vi "Save Message Folder.vi"(8 "error in (no error)":errorcluster, 9 ".proto Path":path, 10 "Output Folder":path) -> (0 "error out":errorcluster)   [LabVIEW 2020, in "LV-Protoc.lvlib" / "LV-Protoc.lvclass"]
uses:
  LV-Protoc.lvclass
  lv-cdm/CDM-Config/Config-JSON/Config-JSON.lvclass
  C:/dev/lv20CE/relink/lv-cdm/CDM-Config/Config Storage/Config Storage.lvclass
  lv-cdm/CDM-Config/Config Element/Write Variant Value.vi
  lv-cdm/CDM-Config/Config Manager/Config Manager.lvclass
  lv-cdm/CDM-Config/Config Element/Config Element.lvclass
  LV-Protoc.lvclass/LV-Protoc.ctl
  lv-cdm/CDM-Config/Config Storage/Config Storage.lvclass
  lv-cdm/CDM-Config/CDM-Config.lvlib
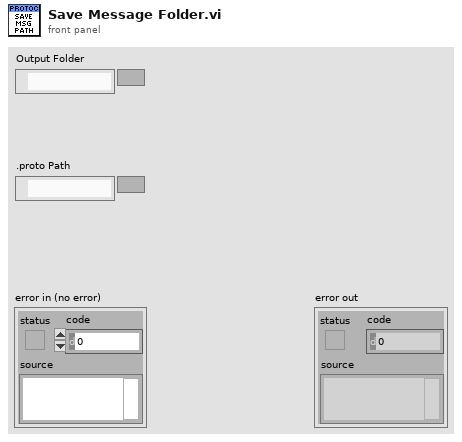
[diagram p1: front panel]
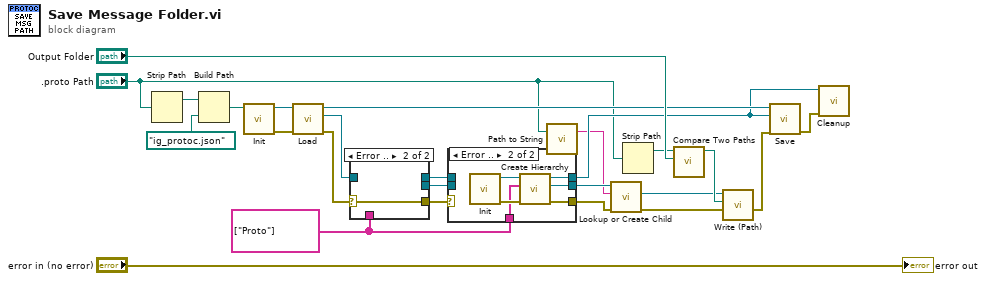
[diagram p0: block diagram]
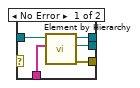
[diagram p2: hidden frame]
diagram:
  w11 = string[] ["Proto"] ("Hierarchy")
  n1 = Strip Path(path=".proto Path") -> (stripped path=w19:path)  [unwired: 1 out]
  n2 = Build Path(base path=w19, name or relative path=path "ig_protoc.json") -> (appended path=w23:path)
  n3 = call "Init.vi"("Path"=w23) -> ("error out"=w22:errorcluster, "Config-JSON out"=w21:refnum<class "Config-JSON.lvclass">)  [unwired: 9 in]
  n4 = call "Load.vi"("error in (no error)"=w22, "Config Storage in"=w21) -> ("error out"=w20:errorcluster, "Config"=w14:refnum<class "Config Manager.lvclass">, "Config Storage out"=w16:refnum<class "Config-JSON.lvclass">)  [unwired: 7 in]
  n5 = case shown="Error .." w20 {
    selector: w20 -> [_ w31]
    tunnel: w14 -> [w30 _]
    tunnel: w11 -> [w29 _]
    tunnel: [w28 _] -> w9
    tunnel: [w27 w31] -> w10
    tunnel: [w26 _] -> w6
    frame No Error {
      n6 = call "Element by Hierarchy.vi"("Hierarchy"=w29, "Config Manager in"=w30) -> ("error out"=w27:errorcluster, "Config Element"=w28:refnum<class "Config Element.lvclass">, "Config Manager out"=w26:refnum<class "Config Manager.lvclass">)  [unwired: 7 in]
    }
    frame Error {
    }
  }
  n7 = case shown="Error .." w10 {
    selector: w10 -> [w33 _]
    tunnel: [w34 w40] -> w13
    tunnel: [w33 w39] -> w12
    tunnel: w11 -> [_ w36]
    tunnel: w9 -> [w34 _]
    tunnel: w6 -> [w32 _]
    tunnel: [w32 w35] -> w5
    frame No Error {
    }
    frame Error {
      n8 = call "Init.vi"() -> ("error out"=w37:errorcluster, "Config Manager out"=w38:refnum<class "Config Manager.lvclass">)  [unwired: 10 in]
      n9 = call "Create Hierarchy.vi"("error in (no error)"=w37, "Hierarchy"=w36, "Config Manager in"=w38) -> ("error out"=w39:errorcluster, "Leaf Element"=w40:refnum<class "Config Element.lvclass">, "Config Manager out"=w35:refnum<class "Config Manager.lvclass">)  [unwired: 6 in]
    }
  }
  n10 = call "Path to String.vi"("Path"=".proto Path") -> ("Path String"=w3:string)  [unwired: 2 in]
  n11 = call "Lookup or Create Child.vi"("error in (no error)"=w12, "Name"=w3, "Config Element in"=w13) -> ("error out"=w7:errorcluster, "Child"=w8:refnum<class "Config Element.lvclass">)  [unwired: 5 in, 2 out]
  n12 = Strip Path(path=".proto Path") -> (stripped path=w4:path)  [unwired: 1 out]
  n13 = call <vilib>:"Compare Two Paths.vi"("Path 2"="Output Folder", "Path 1"=w4) -> ("Relative Path from 1 to 2"=w17:path)  [unwired: 6 in, 3 out]
  n14 = call "Write (Path).vi"("error in (no error)"=w7, "Path Value"=w17, "Config Element in"=w8) -> ("error out"=w15:errorcluster)  [unwired: 7 in, 1 out]
  n15 = call "Save.vi"("error in (no error)"=w15, "Config"=w5, "Config Storage in"=w16) -> ("error out"=w1:errorcluster)  [unwired: 7 in, 1 out]
  n16 = call "Cleanup.vi"("error in (no error)"=w1, "Config Manager in"=w5) -> ()  [unwired: 9 in, 1 out]
  "error out" <- "error in (no error)"
